vi "main.vi"() -> ()   [LabVIEW 2021]
panel:
  out "x1":i32
  out "y1":i32
  out "Len":i32
  out "direction":i32
  out "x":i32
  out "y":i32
  out "index":i32
  out "Numeric":i32
  out "car":i32
  out "valid_dir":i32[][](array[numeric])=[[-1, -1]]
  out "Input":i32[][](array[numeric])=[[0, 2, 3, 2, 1], [1, 0, 0, 3, 1], [2, 1, 3, 3, 1], [3, 3, 1, 2, 1], [4, 5, 0, 3, 1], [5, 1, 0, 2, 2], [6, 3, 0, 2, 2], [7, 1, 2, 2, 2], [8, 3, 3, 3, 2], [9, 4, 4, 2, 2], [10, 2, 5, 2, 2], [11, 4, 5, 2, 2]]
  out "m array":i16[][](array[ring])
  out "Numeric 3":i32
  out "ScanCode":i16
  out "confirm":bool
  out "Numeric 2":i32
  in  "Ring":i32(ring)
  out "Down":bool
  out "Up":bool
  out "Right":bool
  out "Left":bool
  out "reset":bool
  out "init input":i32[][](array[numeric])=[[0, 2, 3, 2, 1], [1, 0, 0, 3, 1], [2, 1, 3, 3, 1], [3, 3, 1, 2, 1], [4, 5, 0, 3, 1], [5, 1, 0, 2, 2], [6, 3, 0, 2, 2], [7, 1, 2, 2, 2], [8, 3, 3, 3, 2], [9, 4, 4, 2, 2], [10, 2, 5, 2, 2], [11, 4, 5, 2, 2]]
  out "Step Counter":i32
  out "win":bool
  in  "stop":bool
  out "orange Down":bool
  out "orange Up":bool
  out "black Down":bool
  out "black Up":bool
  out "Wood Down":bool
  out "Wood Up":bool
  out "grayblue Down":bool
  out "grayblue Up":bool
  out "purple Down":bool
  out "purple Up":bool
  out "Green Right":bool
  out "Green Left":bool
  out "Blue Right":bool
  out "Blue Left":bool
  out "Pink Down":bool
  out "Pink Up":bool
  out "Yellow Right":bool
  out "Yellow Left":bool
  out "tiffany Down":bool
  out "tiffany Up":bool
  out "Brown Right":bool
  out "Brown Left":bool
  out "Red Right":bool
  out "Red Left":bool
  # "Rush Hour (puzzle)"
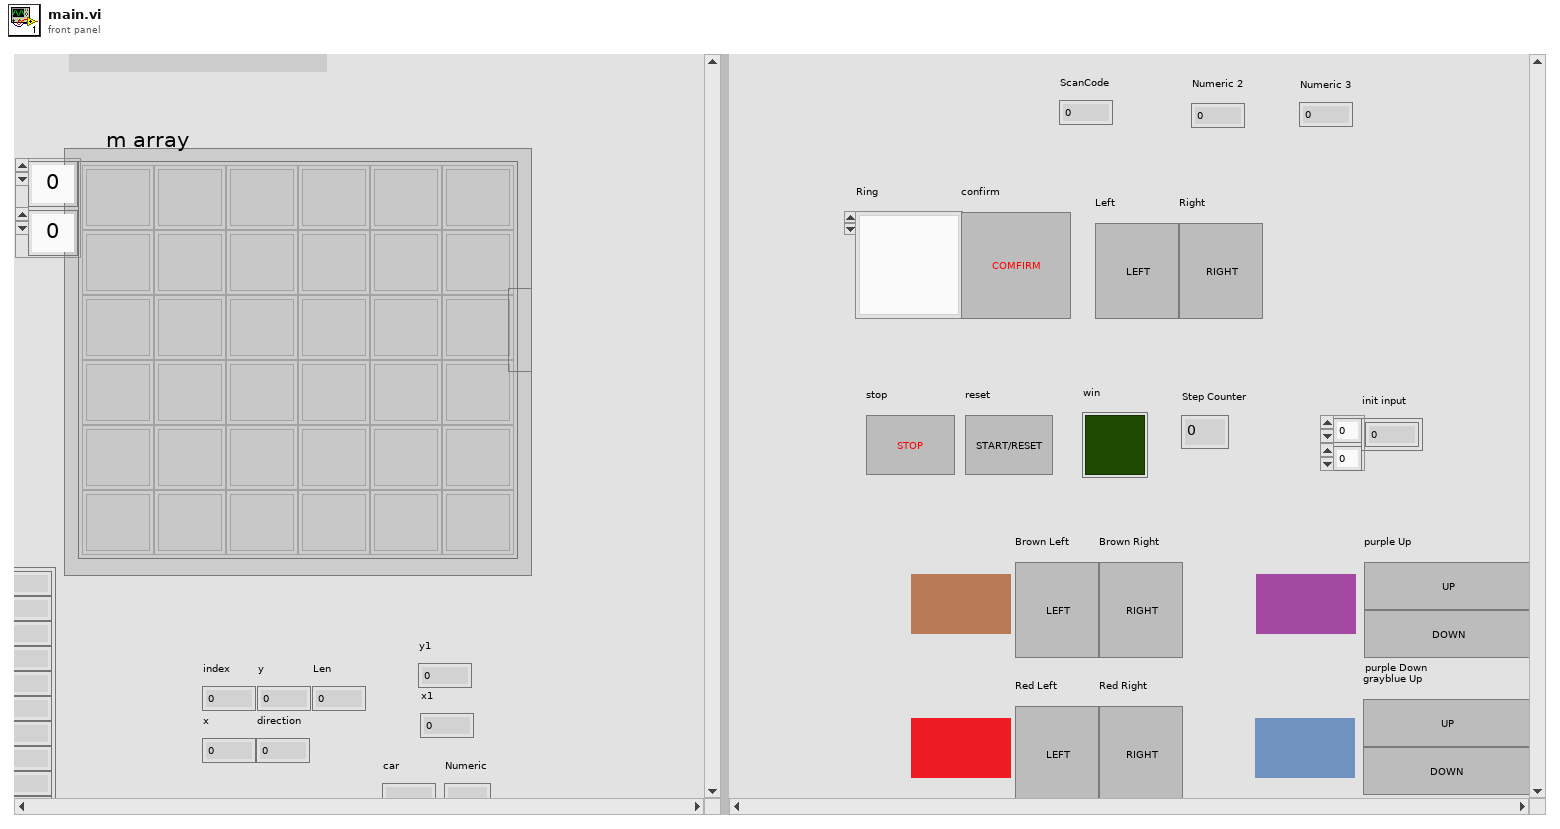
[diagram p1: front panel]
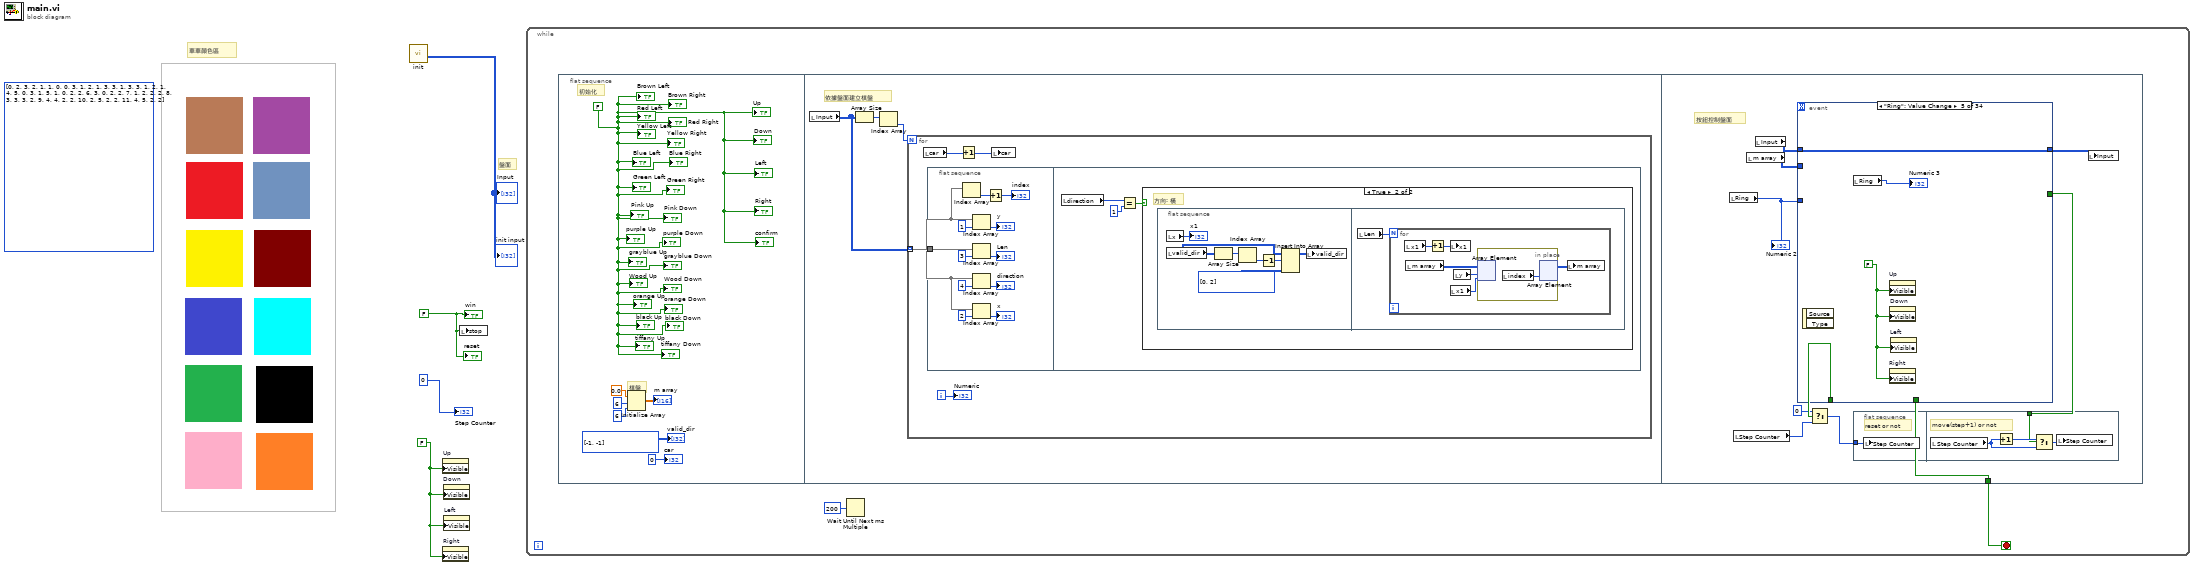
[diagram p0: block diagram]
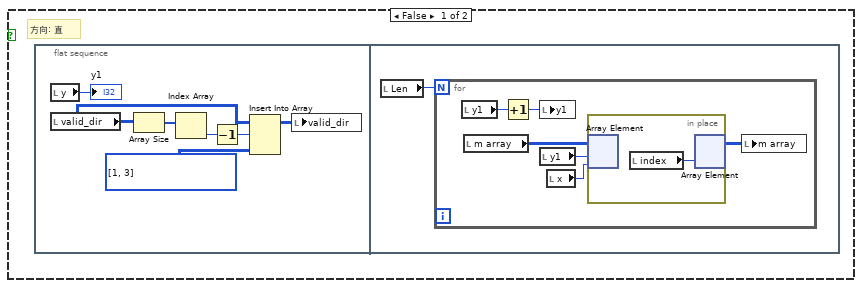
[diagram p2: hidden frame]
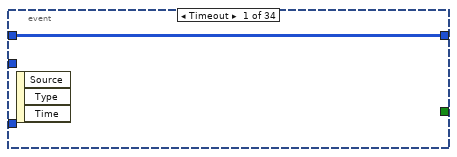
[diagram p3: hidden frame]
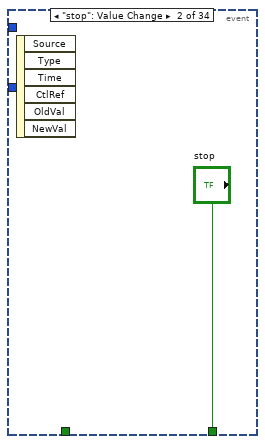
[diagram p4: hidden frame]
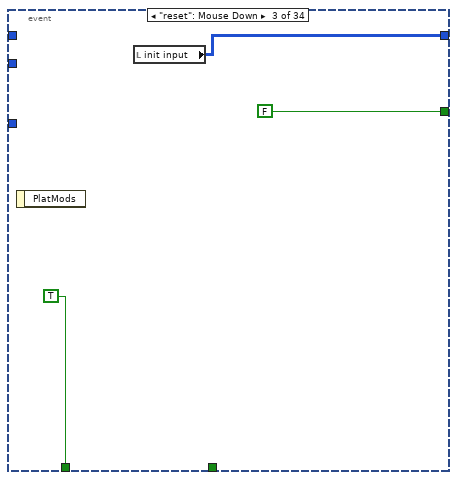
[diagram p5: hidden frame]
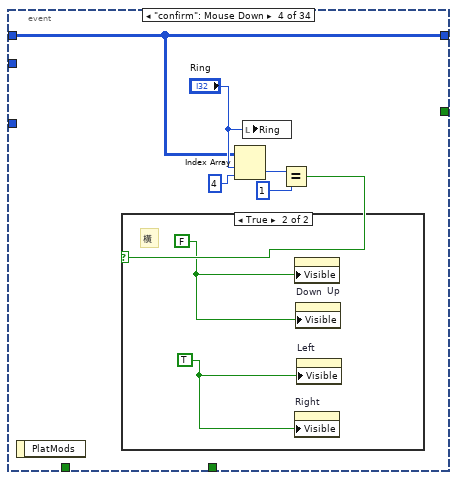
[diagram p6: hidden frame]
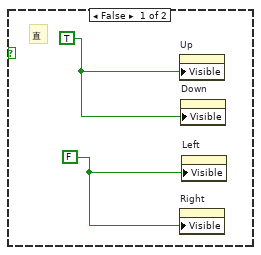
[diagram p7: hidden frame]
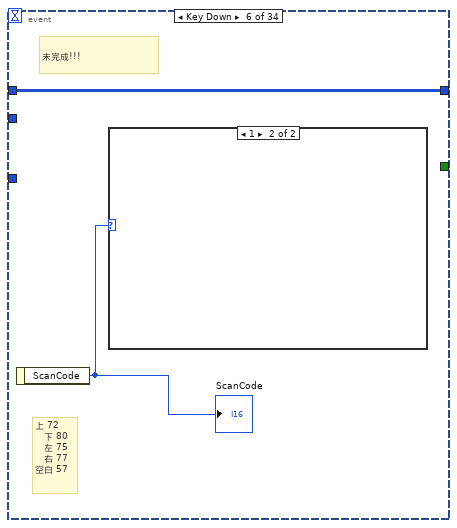
[diagram p8: hidden frame]
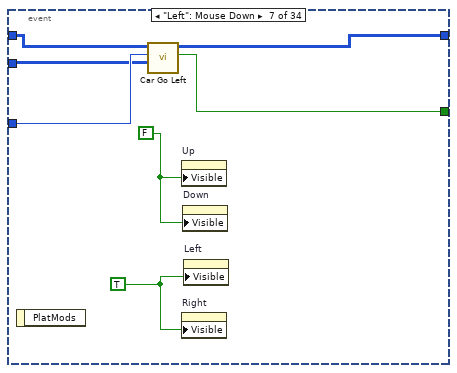
[diagram p10: hidden frame]
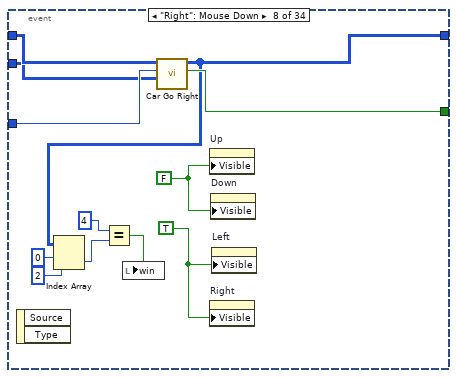
[diagram p11: hidden frame]
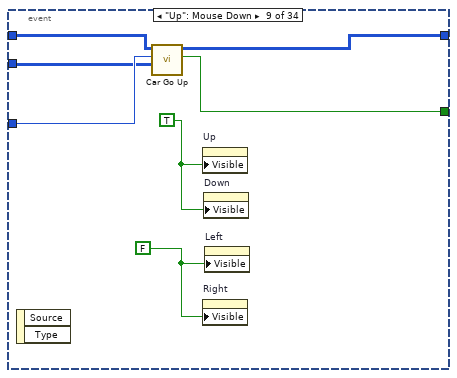
[diagram p12: hidden frame]
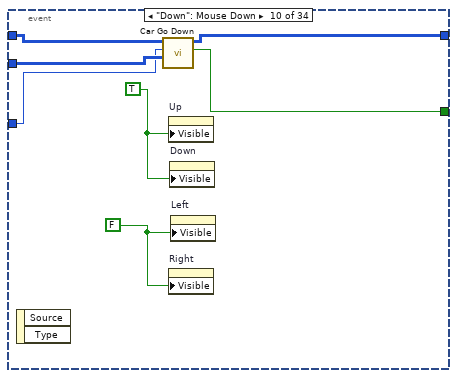
[diagram p13: hidden frame]
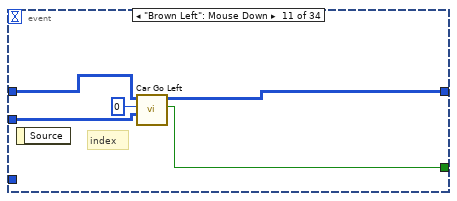
[diagram p14: hidden frame]
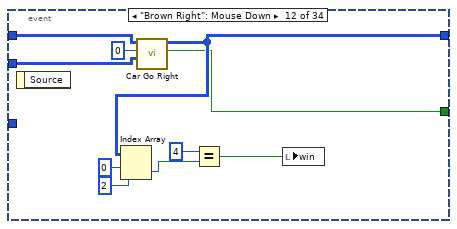
[diagram p15: hidden frame]
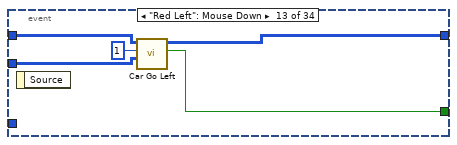
[diagram p16: hidden frame]
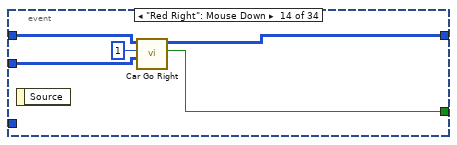
[diagram p17: hidden frame]
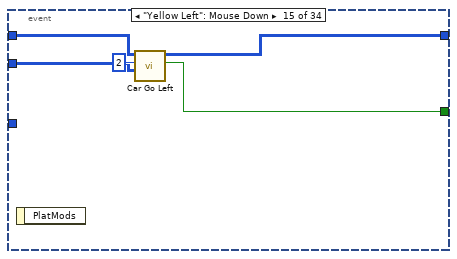
[diagram p18: hidden frame]
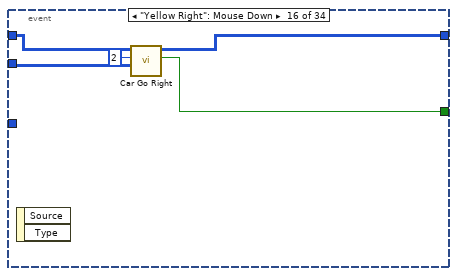
[diagram p19: hidden frame]
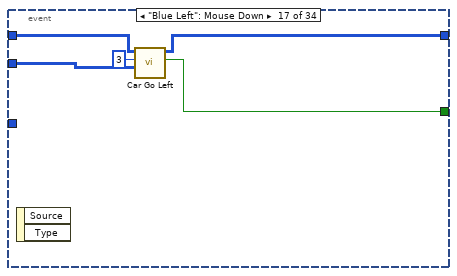
[diagram p20: hidden frame]
diagram:
  w1 = FALSE
  w4 = FALSE
  (unwired) i32[][] [[0, 2, 3, 2, 1], [1, 0, 0, 3, 1], [2, 1, 3, 3, 1], [3, 3, 1, 2, 1], [4, 5, 0, 3, 1], [5, 1, 0, 2, 2], [6, 3, 0, 2, 2], [7, 1, 2, 2, 2], [8, 3, 3, 3, 2], [9, 4, 4, 2, 2], [10, 2, 5, 2, 2], [11, 4, 5, 2, 2]]
  # "盤面"
  # "車車顏色區"
  n1 = call "init.vi"() -> ("Array"=→"Input" →"init input":i32[][])  [unwired: 11 in]
  n2 = property on="Up" class="Bool"("Visible"=w1) -> ()  [unwired: 2 in, 2 out]
  n3 = property on="Right" class="Bool"("Visible"=w1) -> ()  [unwired: 2 in, 2 out]
  n4 = property on="Down" class="Bool"("Visible"=w1) -> ()  [unwired: 2 in, 2 out]
  n5 = property on="Left" class="Bool"("Visible"=w1) -> ()  [unwired: 2 in, 2 out]
  n6 = local write "stop"(w4) -> ()
  n7 = while {
    stop <- w5 stop-if-true
    n8 = flat-sequence {
      tunnel: [w71] -> w5
      frame #0 {
        w7 = FALSE ("Red Left")
        # "初始化"
        # "棋盤"
        n9 = Initialize Array(0.0 ("element"), 6 ("dimension size"), 6 ("dimension size")) -> (→"m array":dbl[][])
        "valid_dir" <- i32[][] [[-1, -1]]
        "car" <- 0
        "Red Right" <- w7
        "Red Left" <- w7
        "Brown Right" <- w7
        "Brown Left" <- w7
        "tiffany Up" <- w7
        "tiffany Down" <- w7
        "Yellow Left" <- w7
        "Yellow Right" <- w7
        "Pink Up" <- w7
        "Pink Down" <- w7
        "Green Right" <- w7
        "Green Left" <- w7
        "Blue Left" <- w7
        "Blue Right" <- w7
        "purple Up" <- w7
        "purple Down" <- w7
        "grayblue Up" <- w7
        "grayblue Down" <- w7
        "Wood Up" <- w7
        "Wood Down" <- w7
        "orange Up" <- w7
        "orange Down" <- w7
        "black Up" <- w7
        "black Down" <- w7
        "Up" <- w7
        "Down" <- w7
        "Left" <- w7
        "Right" <- w7
        "confirm" <- w7
      }
      frame #1 {
        # "依據盤面建立棋盤"
        n10 = local read "Input"() -> (w14:i32[][])
        n11 = Array Size(array=w14) -> (size(s)=w16:i32[])
        n12 = Index Array(array=w16) -> (element=w15:i32)  [unwired: 1 in]
        n13 = for {
          N: w15 -> [_]
          tunnel: w14 -> [w17] mode=indexing
          i -> [w20]
          n14 = local read "car"() -> (w19:i32)
          n15 = flat-sequence {
            tunnel: w17 -> [w21]
            frame #0 {
              n16 = Index Array(array=w21) -> (element=w31:i32)  [unwired: 1 in]
              n17 = Index Array(array=w21, index=1) -> (element=→"y":i32)
              n18 = Index Array(array=w21, index=3) -> (element=→"Len":i32)
              n19 = Index Array(array=w21, index=4) -> (element=→"direction":i32)
              n20 = Index Array(array=w21, index=2) -> (element=→"x":i32)
              n21 = Increment(x=w31) -> (x+1=→"index":i32)
            }
            frame #1 {
              n22 = local read "direction"() -> (w33:i32)
              n23 = Equal?(x=w33, y=1) -> (x = y?=w32:bool)
              n24 = case shown="True" w32 {
                frame False {
                  # "方向: 直"
                  n25 = flat-sequence {
                    frame #0 {
                      n26 = local read "y"() -> (→"y1":i32)
                      n27 = local read "valid_dir"() -> (w41:i32[][])
                      n28 = Array Size(array=w41) -> (size(s)=w40:i32[])
                      n29 = Index Array(array=w40) -> (element=w38:i32)  [unwired: 1 in]
                      n30 = Decrement(x=w38) -> (x-1=w39:i32)
                      n31 = Insert Into Array(array=w41, index (row)=w39, new element=i32[][] [[1, 3]]) -> (w37:i32[][])  [unwired: 1 in]
                      n32 = local write "valid_dir"(w37) -> ()
                    }
                    frame #1 {
                      n33 = local read "Len"() -> (w42:i32)
                      n34 = for {
                        N: w42 -> [_]
                        n35 = local read "y1"() -> (w44:i32)
                        n36 = local read "m array"() -> (w48:i16[][])
                        n37 = Increment(x=w44) -> (x+1=w43:i32)
                        n38 = local write "y1"(w43) -> ()
                        n39 = local read "y1"() -> (w47:i32)
                        n40 = local read "x"() -> (w46:i32)
                        n41 = in-place {
                          n42 = in-place-array #1(w48, w47, w46) -> ()  [unwired: 1 out]
                          n43 = local read "index"() -> (w49:i32)
                          n44 = in-place-array #1(w49) -> (w45:i16[][])  [unwired: 2 out]
                        }
                        n45 = local write "m array"(w45) -> ()
                      }
                    }
                  }
                }
                frame True {
                  # "方向: 橫"
                  n46 = flat-sequence {
                    frame #0 {
                      n47 = local read "x"() -> (→"x1":i32)
                      n48 = local read "valid_dir"() -> (w55:i32[][])
                      n49 = Array Size(array=w55) -> (size(s)=w54:i32[])
                      n50 = Index Array(array=w54) -> (element=w52:i32)  [unwired: 1 in]
                      n51 = Decrement(x=w52) -> (x-1=w53:i32)
                      n52 = Insert Into Array(array=w55, index (row)=w53, new element=i32[][] [[0, 2]]) -> (w51:i32[][])  [unwired: 1 in]
                      n53 = local write "valid_dir"(w51) -> ()
                    }
                    frame #1 {
                      n54 = local read "Len"() -> (w57:i32)
                      n55 = for {
                        N: w57 -> [_]
                        n56 = local read "x1"() -> (w59:i32)
                        n57 = local read "m array"() -> (w63:i16[][])
                        n58 = Increment(x=w59) -> (x+1=w58:i32)
                        n59 = local write "x1"(w58) -> ()
                        n60 = local read "x1"() -> (w61:i32)
                        n61 = local read "y"() -> (w62:i32)
                        n62 = in-place {
                          n63 = in-place-array #2(w63, w62, w61) -> ()  [unwired: 1 out]
                          n64 = local read "index"() -> (w64:i32)
                          n65 = in-place-array #2(w64) -> (w60:i16[][])  [unwired: 2 out]
                        }
                        n66 = local write "m array"(w60) -> ()
                      }
                    }
                  }
                }
              }
            }
          }
          n67 = Increment(x=w19) -> (x+1=w18:i32)
          n68 = local write "car"(w18) -> ()
          "Numeric" <- w20
        }
      }
      frame #2 {
        # "按鈕控制盤面"
        n69 = local read "Ring"() -> (w65:i32)
        "Numeric 2" <- w65
        n70 = local read "Step Counter"() -> (w67:i32)
        n71 = local read "m array"() -> (w73:i16[][])
        n72 = local read "Input"() -> (w74:i32[][])
        n73 = event shown="[4] \"Ring\": Value Change" {
          selector: _ -> [_ _ _ _ _ _ _ _ _ _ _ _ _ _ _ _ _ _ _ _ _ _ _ _ _ _ _ _ _ _ _ _ _ _]
          dyn-events: _ -> [_ _ _ _ _ _ _ _ _ _ _ _ _ _ _ _ _ _ _ _ _ _ _ _ _ _ _ _ _ _ _ _ _ _]
          timeout: _ -> [_ _ _ _ _ _ _ _ _ _ _ _ _ _ _ _ _ _ _ _ _ _ _ _ _ _ _ _ _ _ _ _ _ _]
          tunnel: w74 -> [w80 _ _ w85 w97 w99 w106 w118 w125 w132 w135 w146 w151 w155 w161 w167 w171 w176 w181 w186 w192 w197 w201 w206 w211 w216 w221 w226 w231 w236 w241 w246 w251 w256]
          tunnel: w73 -> [_ _ _ _ _ _ w104 w116 w123 w131 w136 w145 w150 w156 w160 w166 w170 w175 w180 w185 w191 w196 w200 w205 w210 w215 w220 w225 w230 w235 w240 w245 w250 w255]
          tunnel: [w80 _ w84 w85 w97 w99 w102 w109 w121 w128 w134 w144 w149 w154 w159 w164 w169 w174 w179 w184 w190 w195 w199 w204 w209 w214 w219 w224 w229 w234 w239 w244 w249 w254] -> w72
          tunnel: [_ "stop" _ _ _ _ _ _ _ _ _ _ _ _ _ _ _ _ _ _ _ _ _ _ _ _ _ _ _ _ _ _ _ _] -> w71
          tunnel: [_ _ FALSE _ _ _ w103 w115 w122 w129 w133 w138 w148 w153 w158 w163 w168 w173 w178 w183 w188 w193 w198 w203 w208 w213 w218 w223 w228 w233 w238 w243 w248 w253] -> w70
          tunnel: [_ _ TRUE _ _ _ _ _ _ _ _ _ _ _ _ _ _ _ _ _ _ _ _ _ _ _ _ _ _ _ _ _ _ _] -> w68
          tunnel: w65 -> [_ _ _ _ _ _ w105 w117 w124 w130 _ _ _ _ _ _ _ _ _ _ _ _ _ _ _ _ _ _ _ _ _ _ _ _]
          event Timeout {
            n74 = event-data() -> ()  [unwired: 1 in, 3 out]
          }
          event "stop": Value Change {
            n75 = event-data() -> ()  [unwired: 1 in, 6 out]
          }
          event "reset": Mouse Down {
            n76 = event-data() -> ()  [unwired: 1 in, 1 out]
            n77 = local read "init input"() -> (w84:i32[][])
          }
          event "confirm": Mouse Down {
            n78 = event-data() -> ()  [unwired: 1 in, 1 out]
            n79 = Index Array(array=w85, index (row)="Ring", index (col)=4) -> (element=w88:i32)
            n80 = local write "Ring"("Ring") -> ()
            n81 = Equal?(x=w88, y=1) -> (x = y?=w86:bool)
            n82 = case shown="True" w86 {
              frame False {
                w91 = FALSE
                w92 = TRUE
                # "直"
                n83 = property on="Up" class="Bool"("Visible"=w92) -> ()  [unwired: 2 in, 2 out]
                n84 = property on="Right" class="Bool"("Visible"=w91) -> ()  [unwired: 2 in, 2 out]
                n85 = property on="Down" class="Bool"("Visible"=w92) -> ()  [unwired: 2 in, 2 out]
                n86 = property on="Left" class="Bool"("Visible"=w91) -> ()  [unwired: 2 in, 2 out]
              }
              frame True {
                w94 = TRUE
                w93 = FALSE
                # "橫"
                n87 = property on="Up" class="Bool"("Visible"=w93) -> ()  [unwired: 2 in, 2 out]
                n88 = property on="Right" class="Bool"("Visible"=w94) -> ()  [unwired: 2 in, 2 out]
                n89 = property on="Down" class="Bool"("Visible"=w93) -> ()  [unwired: 2 in, 2 out]
                n90 = property on="Left" class="Bool"("Visible"=w94) -> ()  [unwired: 2 in, 2 out]
              }
            }
          }
          event "Ring": Value Change {
            w96 = FALSE
            n91 = event-data() -> ()  [unwired: 1 in, 2 out]
            n92 = local read "Ring"() -> (→"Numeric 3":i32)
            n93 = property on="Up" class="Bool"("Visible"=w96) -> ()  [unwired: 2 in, 2 out]
            n94 = property on="Right" class="Bool"("Visible"=w96) -> ()  [unwired: 2 in, 2 out]
            n95 = property on="Down" class="Bool"("Visible"=w96) -> ()  [unwired: 2 in, 2 out]
            n96 = property on="Left" class="Bool"("Visible"=w96) -> ()  [unwired: 2 in, 2 out]
          }
          event Key Down {
            # "未完成!!!"
            # "上 72\n　下 80\n　左 75\n　右 77\n空白 57"
            n97 = event-data() -> ("ScanCode"=w98:i16)  [unwired: 1 in]
            "ScanCode" <- w98
            n98 = case shown="1" w98 {
              frame 0, Default {
              }
              frame 1 {
              }
            }
          }
          event "Left": Mouse Down {
            w100 = TRUE ("Visible")
            w101 = FALSE
            n99 = event-data() -> ()  [unwired: 1 in, 1 out]
            n100 = call "Car Go Left.vi"("m array"=w104, "Numeric"=w105, "Input in"=w106) -> ("move or not"=w103:bool, "Input out"=w102:i32[][])  [unwired: 7 in]
            n101 = property on="Up" class="Bool"("Visible"=w101) -> ()  [unwired: 2 in, 2 out]
            n102 = property on="Right" class="Bool"("Visible"=w100) -> ()  [unwired: 2 in, 2 out]
            n103 = property on="Down" class="Bool"("Visible"=w101) -> ()  [unwired: 2 in, 2 out]
            n104 = property on="Left" class="Bool"("Visible"=w100) -> ()  [unwired: 2 in, 2 out]
          }
          event "Right": Mouse Down {
            w107 = TRUE
            w114 = FALSE
            n105 = event-data() -> ()  [unwired: 1 in, 2 out]
            n106 = call "Car Go Right.vi"("m array"=w116, "Numeric"=w117, "Input in"=w118) -> ("move or not"=w115:bool, "Input out"=w109:i32[][])  [unwired: 7 in]
            n107 = Index Array(array=w109, index (row)=0, index (col)=2 ("disabled index (col)")) -> (element=w113:i32)
            n108 = Equal?(x=4, y=w113) -> (x = y?=w112:bool)
            n109 = local write "win"(w112) -> ()
            n110 = property on="Up" class="Bool"("Visible"=w114) -> ()  [unwired: 2 in, 2 out]
            n111 = property on="Right" class="Bool"("Visible"=w107) -> ()  [unwired: 2 in, 2 out]
            n112 = property on="Down" class="Bool"("Visible"=w114) -> ()  [unwired: 2 in, 2 out]
            n113 = property on="Left" class="Bool"("Visible"=w107) -> ()  [unwired: 2 in, 2 out]
          }
          event "Up": Mouse Down {
            w119 = FALSE
            w120 = TRUE
            n114 = event-data() -> ()  [unwired: 1 in, 2 out]
            n115 = call "Car Go Up.vi"("m array"=w123, "Numeric"=w124, "Input in"=w125) -> ("move or not"=w122:bool, "Input out"=w121:i32[][])  [unwired: 7 in]
            n116 = property on="Up" class="Bool"("Visible"=w120) -> ()  [unwired: 2 in, 2 out]
            n117 = property on="Right" class="Bool"("Visible"=w119) -> ()  [unwired: 2 in, 2 out]
            n118 = property on="Down" class="Bool"("Visible"=w120) -> ()  [unwired: 2 in, 2 out]
            n119 = property on="Left" class="Bool"("Visible"=w119) -> ()  [unwired: 2 in, 2 out]
          }
          event "Down": Mouse Down {
            w126 = FALSE
            w127 = TRUE
            n120 = event-data() -> ()  [unwired: 1 in, 2 out]
            n121 = call "Car Go Down.vi"("m array"=w131, "Numeric"=w130, "Input in"=w132) -> ("move or not"=w129:bool, "Input out"=w128:i32[][])  [unwired: 7 in]
            n122 = property on="Up" class="Bool"("Visible"=w127) -> ()  [unwired: 2 in, 2 out]
            n123 = property on="Right" class="Bool"("Visible"=w126) -> ()  [unwired: 2 in, 2 out]
            n124 = property on="Down" class="Bool"("Visible"=w127) -> ()  [unwired: 2 in, 2 out]
            n125 = property on="Left" class="Bool"("Visible"=w126) -> ()  [unwired: 2 in, 2 out]
          }
          event "Brown Left": Mouse Down {
            # "index"
            n126 = event-data() -> ()  [unwired: 1 in, 1 out]
            n127 = call "Car Go Left.vi"("m array"=w136, "Numeric"=0, "Input in"=w135) -> ("move or not"=w133:bool, "Input out"=w134:i32[][])  [unwired: 7 in]
          }
          event "Brown Right": Mouse Down {
            n128 = event-data() -> ()  [unwired: 1 in, 1 out]
            n129 = call "Car Go Right.vi"("m array"=w145, "Numeric"=0, "Input in"=w146) -> ("move or not"=w138:bool, "Input out"=w144:i32[][])  [unwired: 7 in]
            n130 = Index Array(array=w144, index (row)=0, index (col)=2 ("disabled index (col)")) -> (element=w141:i32)
            n131 = Equal?(x=4, y=w141) -> (x = y?=w139:bool)
            n132 = local write "win"(w139) -> ()
          }
          event "Red Left": Mouse Down {
            n133 = event-data() -> ()  [unwired: 1 in, 1 out]
            n134 = call "Car Go Left.vi"("m array"=w150, "Numeric"=1, "Input in"=w151) -> ("move or not"=w148:bool, "Input out"=w149:i32[][])  [unwired: 7 in]
          }
          event "Red Right": Mouse Down {
            n135 = event-data() -> ()  [unwired: 1 in, 1 out]
            n136 = call "Car Go Right.vi"("m array"=w156, "Numeric"=1, "Input in"=w155) -> ("move or not"=w153:bool, "Input out"=w154:i32[][])  [unwired: 7 in]
          }
          event "Yellow Left": Mouse Down {
            n137 = event-data() -> ()  [unwired: 1 in, 1 out]
            n138 = call "Car Go Left.vi"("m array"=w160, "Numeric"=2, "Input in"=w161) -> ("move or not"=w158:bool, "Input out"=w159:i32[][])  [unwired: 7 in]
          }
          event "Yellow Right": Mouse Down {
            n139 = event-data() -> ()  [unwired: 1 in, 2 out]
            n140 = call "Car Go Right.vi"("m array"=w166, "Numeric"=2, "Input in"=w167) -> ("move or not"=w163:bool, "Input out"=w164:i32[][])  [unwired: 7 in]
          }
          event "Blue Left": Mouse Down {
            n141 = event-data() -> ()  [unwired: 1 in, 2 out]
            n142 = call "Car Go Left.vi"("m array"=w170, "Numeric"=3, "Input in"=w171) -> ("move or not"=w168:bool, "Input out"=w169:i32[][])  [unwired: 7 in]
          }
          event "Blue Right": Mouse Down {
            n143 = event-data() -> ()  [unwired: 1 in, 2 out]
            n144 = call "Car Go Right.vi"("m array"=w175, "Numeric"=3, "Input in"=w176) -> ("move or not"=w173:bool, "Input out"=w174:i32[][])  [unwired: 7 in]
          }
          event "Green Left": Mouse Down {
            n145 = event-data() -> ()  [unwired: 1 in, 2 out]
            n146 = call "Car Go Left.vi"("m array"=w180, "Numeric"=4, "Input in"=w181) -> ("move or not"=w178:bool, "Input out"=w179:i32[][])  [unwired: 7 in]
          }
          event "Green Right": Mouse Down {
            n147 = event-data() -> ()  [unwired: 1 in, 2 out]
            n148 = call "Car Go Right.vi"("m array"=w185, "Numeric"=4, "Input in"=w186) -> ("move or not"=w183:bool, "Input out"=w184:i32[][])  [unwired: 7 in]
          }
          event "Pink Up": Mouse Down {
            n149 = event-data() -> ()  [unwired: 1 in, 2 out]
            n150 = call "Car Go Up.vi"("m array"=w191, "Numeric"=5, "Input in"=w192) -> ("move or not"=w188:bool, "Input out"=w190:i32[][])  [unwired: 7 in]
          }
          event "Pink Down": Mouse Down {
            n151 = event-data() -> ()  [unwired: 1 in, 2 out]
            n152 = call "Car Go Down.vi"("m array"=w196, "Numeric"=5, "Input in"=w197) -> ("move or not"=w193:bool, "Input out"=w195:i32[][])  [unwired: 7 in]
          }
          event "purple Up": Mouse Down {
            n153 = event-data() -> ()  [unwired: 1 in, 2 out]
            n154 = call "Car Go Up.vi"("m array"=w200, "Numeric"=6, "Input in"=w201) -> ("move or not"=w198:bool, "Input out"=w199:i32[][])  [unwired: 7 in]
          }
          event "purple Down": Mouse Down {
            n155 = event-data() -> ()  [unwired: 1 in, 2 out]
            n156 = call "Car Go Down.vi"("m array"=w205, "Numeric"=6, "Input in"=w206) -> ("move or not"=w203:bool, "Input out"=w204:i32[][])  [unwired: 7 in]
          }
          event "grayblue Up": Mouse Down {
            n157 = event-data() -> ()  [unwired: 1 in, 2 out]
            n158 = call "Car Go Up.vi"("m array"=w210, "Numeric"=7, "Input in"=w211) -> ("move or not"=w208:bool, "Input out"=w209:i32[][])  [unwired: 7 in]
          }
          event "grayblue Down": Mouse Down {
            n159 = event-data() -> ()  [unwired: 1 in, 2 out]
            n160 = call "Car Go Down.vi"("m array"=w215, "Numeric"=7, "Input in"=w216) -> ("move or not"=w213:bool, "Input out"=w214:i32[][])  [unwired: 7 in]
          }
          event "Wood Up": Mouse Down {
            n161 = event-data() -> ()  [unwired: 1 in, 2 out]
            n162 = call "Car Go Up.vi"("m array"=w220, "Numeric"=8, "Input in"=w221) -> ("move or not"=w218:bool, "Input out"=w219:i32[][])  [unwired: 7 in]
          }
          event "Wood Down": Mouse Down {
            n163 = event-data() -> ()  [unwired: 1 in, 2 out]
            n164 = call "Car Go Down.vi"("m array"=w225, "Numeric"=8, "Input in"=w226) -> ("move or not"=w223:bool, "Input out"=w224:i32[][])  [unwired: 7 in]
          }
          event "tiffany Up": Mouse Down {
            # "index"
            n165 = event-data() -> ()  [unwired: 1 in, 1 out]
            n166 = call "Car Go Up.vi"("m array"=w230, "Numeric"=9, "Input in"=w231) -> ("move or not"=w228:bool, "Input out"=w229:i32[][])  [unwired: 7 in]
          }
          event "tiffany Down": Mouse Down {
            # "index"
            n167 = event-data() -> ()  [unwired: 1 in, 1 out]
            n168 = call "Car Go Down.vi"("m array"=w235, "Numeric"=9, "Input in"=w236) -> ("move or not"=w233:bool, "Input out"=w234:i32[][])  [unwired: 7 in]
          }
          event "black Up": Mouse Down {
            n169 = event-data() -> ()  [unwired: 1 in, 1 out]
            n170 = call "Car Go Up.vi"("m array"=w240, "Numeric"=10, "Input in"=w241) -> ("move or not"=w238:bool, "Input out"=w239:i32[][])  [unwired: 7 in]
          }
          event "black Down": Mouse Down {
            n171 = event-data() -> ()  [unwired: 1 in, 3 out]
            n172 = call "Car Go Down.vi"("m array"=w245, "Numeric"=10, "Input in"=w246) -> ("move or not"=w243:bool, "Input out"=w244:i32[][])  [unwired: 7 in]
          }
          event "orange Up": Mouse Down {
            n173 = event-data() -> ()  [unwired: 1 in, 1 out]
            n174 = call "Car Go Up.vi"("m array"=w250, "Numeric"=11, "Input in"=w251) -> ("move or not"=w248:bool, "Input out"=w249:i32[][])  [unwired: 7 in]
          }
          event "orange Down": Mouse Down {
            n175 = event-data() -> ()  [unwired: 1 in, 1 out]
            n176 = call "Car Go Down.vi"("m array"=w255, "Numeric"=11, "Input in"=w256) -> ("move or not"=w253:bool, "Input out"=w254:i32[][])  [unwired: 7 in]
          }
        }
        n177 = Select(t=0 ("Step Counter"), s=w68, f=w67) -> (s? t:f=w69:i32)
        n178 = flat-sequence {
          tunnel: w69 -> [w75]
          tunnel: w70 -> [w77]
          frame #0 {
            # "reset or not"
            n179 = local write "Step Counter"(w75) -> ()
          }
          frame #1 {
            # "move(step+1) or not"
            n180 = local read "Step Counter"() -> (w76:i32)
            n181 = Increment(x=w76) -> (x+1=w78:i32)
            n182 = Select(t=w78, s=w77, f=w76) -> (s? t:f=w79:i32)
            n183 = local write "Step Counter"(w79) -> ()
          }
        }
        n184 = local write "Input"(w72) -> ()
      }
    }
    n185 = Wait Until Next ms Multiple(millisecond multiple=u32 200 ("millisecond timer value")) -> ()  [unwired: 1 out]
  }
  "win" <- w4
  "reset" <- w4
  "Step Counter" <- 0
